vi "rqcBob Configure.vi"   [LabVIEW 2019, in "rqcBob.lvclass"]
uses:
  rqcBob.lvclass
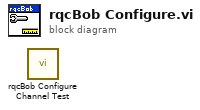
[diagram p0: block diagram]
diagram:
  n1 = call "rqcBob Configure Channel Test.vi"() -> ()  [unwired: 14 in, 2 out]
